vi "main.vi"() -> ()   [LabVIEW 2019]
uses:
  ServerCommands.ctl
  <vilib>/ErrorRing/Error Ring.xnode
panel:
  out "Log":string
  in  "stop":bool
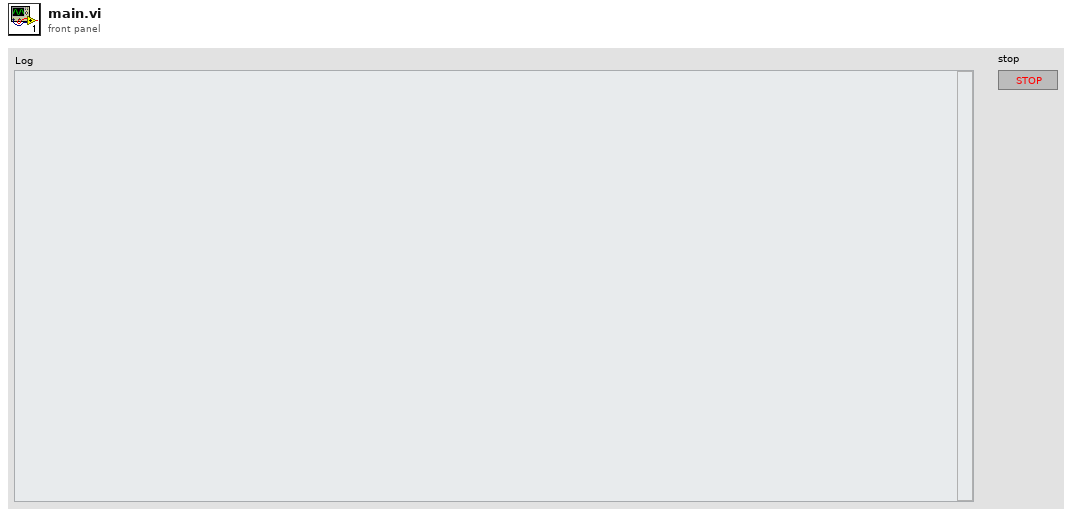
[diagram p1: front panel]
types:
  T1 = typedef "ServerCommands.ctl" = enum16{"Initialize", "Listen", "Run"}
  T2 = enum16{"Standard", "Buffered", "CRLF", "Immediate"}
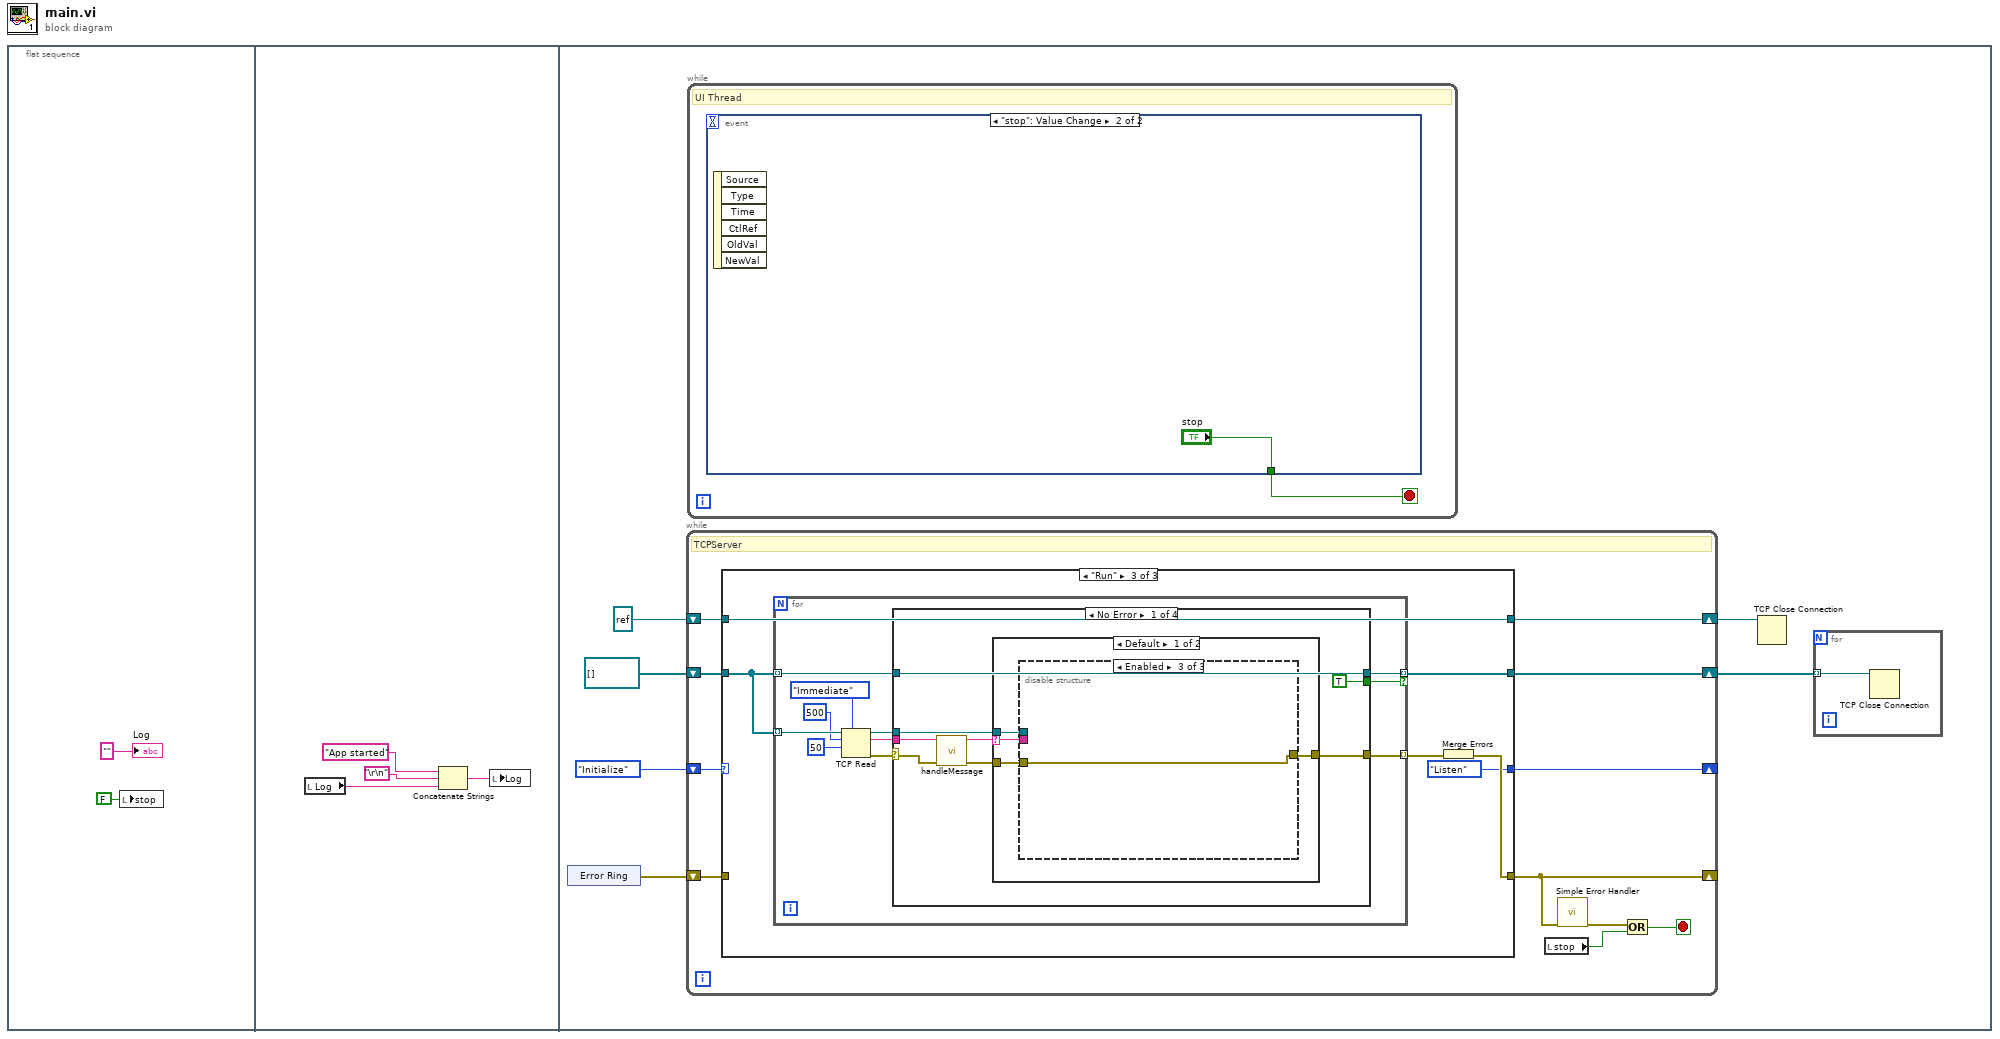
[diagram p0: block diagram]
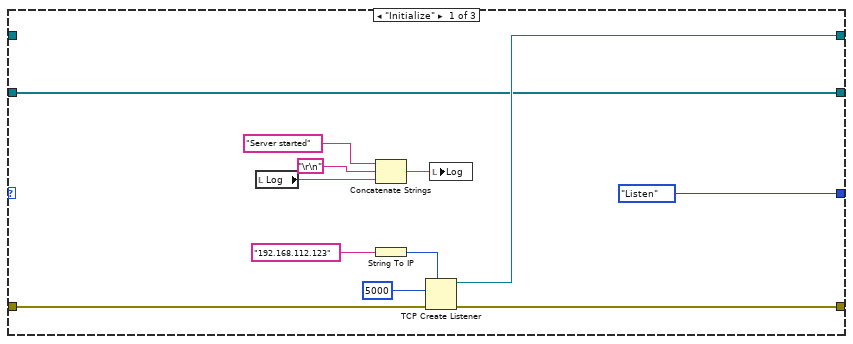
[diagram p2: hidden frame]
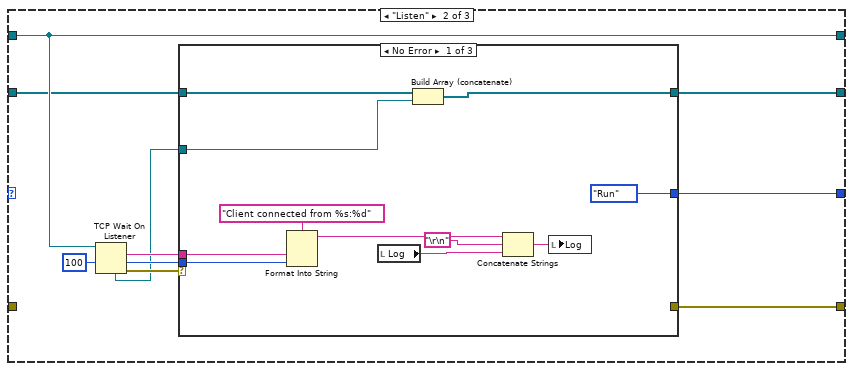
[diagram p3: hidden frame]
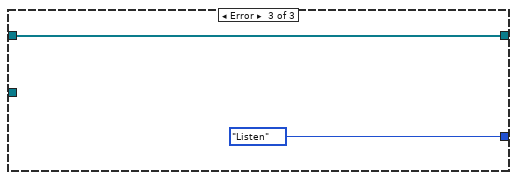
[diagram p5: hidden frame]
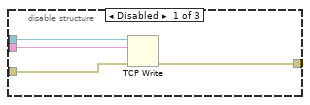
[diagram p6: hidden frame]
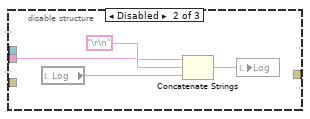
[diagram p7: hidden frame]
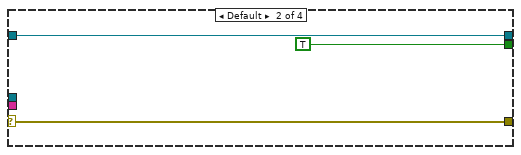
[diagram p9: hidden frame]
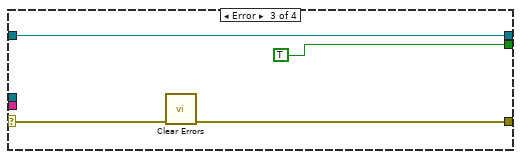
[diagram p10: hidden frame]
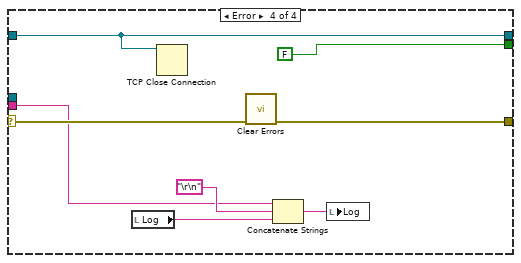
[diagram p11: hidden frame]
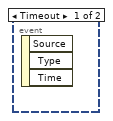
[diagram p12: hidden frame]
diagram:
  n1 = flat-sequence {
    frame #0 {
      n2 = local write "stop"(FALSE ("stop")) -> ()
      "Log" <- ""
    }
    frame #1 {
      n3 = local read "Log"() -> (w6:string)
      n4 = Concatenate Strings("App started" ("string"), "\r\n", w6) -> (w5:string)
      n5 = local write "Log"(w5) -> ()
    }
    frame #2 {
      n6 = xnode "Error Ring"() -> ("error out"=w11:errorcluster)
      n7 = while {
        shift-right: [w20] -> _
        shift-left: w11 -> [w24]
        shift-right: [w22] -> w8
        shift-left: refnum<k5> refnum ("listener ID") -> [w23]
        shift-right: [w21] -> _
        shift-left: ServerCommands."Initialize" ("ServerCommands") -> [w25]
        shift-right: [w15] -> w7
        shift-left: refnum<k5>[] [] -> [w16]
        stop <- w17 stop-if-true
        # "TCPServer"
        n8 = case shown="\"Run\"" w25 {
          tunnel: w24 -> [w33 _ _]
          tunnel: [w34 w43 w67] -> w20
          tunnel: [w32 w47 w68] -> w22
          tunnel: w23 -> [_ w47 w68]
          tunnel: [ServerCommands."Listen" ("ServerCommands") w41 ServerCommands."Listen" ("ServerCommands")] -> w21
          tunnel: w16 -> [w26 w40 w65]
          tunnel: [w26 w39 w64] -> w15
          frame "Initialize" {
            n9 = local read "Log"() -> (w29:string)
            n10 = Concatenate Strings("Server started" ("string"), "\r\n", w29) -> (w27:string)
            n11 = String To IP(1:"192.168.112.123" ("name")) -> (0:w37:u32)
            n12 = TCP Create Listener(7:w37, 8:w33, 10:u16 5000 ("port")) -> (0:w34:errorcluster, 3:w32:refnum<k5>)  [unwired: 2 in, 1 out]
            n13 = local write "Log"(w27) -> ()
          }
          frame "Listen" {
            n14 = TCP Wait On Listener(9:100 ("timeout ms (wait forever: -1)"), 11:w47) -> (0:w46:errorcluster, 1:w44:u16, 2:w45:string, 4:w38:refnum<k5>)  [unwired: 2 in, 1 out]
            n15 = case shown="No Error" w46 {
              selector: w46 -> [_ w60 _]
              tunnel: w38 -> [w49 _ _]
              tunnel: w45 -> [w54 _ _]
              tunnel: w44 -> [w53 _ _]
              tunnel: [_ w60 _] -> w43
              tunnel: [ServerCommands."Run" ("ServerCommands") _ ServerCommands."Listen" ("ServerCommands")] -> w41
              tunnel: w40 -> [w50 w59 w61]
              tunnel: [w48 w59 w61] -> w39
              frame No Error {
                n16 = Format Into String(format string="Client connected from %s:%d", w54, w53) -> (resulting string=w52:string)  [unwired: 2 in, 1 out]
                n17 = local read "Log"() -> (w56:string)
                n18 = Build Array (concatenate)(w50, w49) -> (w48:refnum<k5>[])
                n19 = Concatenate Strings(w52, "\r\n", w56) -> (w57:string)
                n20 = local write "Log"(w57) -> ()
              }
              frame Default {
              }
              frame Error {
              }
            }
          }
          frame "Run" {
            n21 = for {
              tunnel: w65 -> [w79] mode=indexing
              tunnel: [w74] -> w66 mode=indexing
              tunnel: w65 -> [w73] mode=indexing
              tunnel: [w72] -> w64 mode=indexing if=w71
              n22 = TCP Read(connection ID=w79, bytes to read=500, 7:T2."Immediate" ("mode (standard)"), 9:50 ("timeout ms (25000)")) -> (connection ID out=w75:refnum<k5>, data out=w76:string, error out=w77:errorcluster)  [unwired: 1 in]
              n23 = case shown="No Error" w77 {
                selector: w77 -> [w86 w104 w108 w116]
                tunnel: w76 -> [w87 _ _ w109]
                tunnel: w75 -> [w83 _ _ _]
                tunnel: [w82 w104 w107 w115] -> w74
                tunnel: w73 -> [w81 w103 w106 w113]
                tunnel: [w81 w103 w106 w113] -> w72
                tunnel: [TRUE TRUE TRUE FALSE] -> w71
                frame No Error {
                  n24 = call "handleMessage.vi"("error in (no error)"=w86, "InputMessage"=w87) -> ("error out"=w84:errorcluster, "OutputMessage"=w85:string)  [unwired: 8 in]
                  n25 = case shown="Default" w85 {
                    selector: w85 -> [w90 _]
                    tunnel: w84 -> [w89 w101]
                    tunnel: w83 -> [w91 _]
                    tunnel: [w88 w101] -> w82
                    frame Default {
                      n26 = disable-structure shown="Enabled" {
                        disable-tunnel: w91 -> [w95 _ _]
                        disable-tunnel: w90 -> [w94 w96 _]
                        disable-tunnel: w89 -> [w93 _ w100]
                        disable-tunnel: [w92 _ w100] -> w88
                        frame Disabled {
                          n27 = TCP Write(connection ID=w95, data in=w94, error in (no error)=w93) -> (error out=w92:errorcluster)  [unwired: 1 in, 2 out]
                        }
                        frame Disabled {
                          n28 = local read "Log"() -> (w97:string)
                          n29 = Concatenate Strings(w96, "\r\n", w97) -> (w98:string)
                          n30 = local write "Log"(w98) -> ()
                        }
                        frame Enabled {
                        }
                      }
                    }
                    frame "" {
                    }
                  }
                }
                frame Default {
                }
                frame Error {
                  n31 = call <vilib>:"Clear Errors.vi"("error in (no error)"=w108) -> ("error out"=w107:errorcluster)  [unwired: 5 in, 1 out]
                }
                frame Error {
                  n32 = local read "Log"() -> (w111:string)
                  n33 = TCP Close Connection(connection ID=w113) -> ()  [unwired: 2 in, 2 out]
                  n34 = call <vilib>:"Clear Errors.vi"("error in (no error)"=w116) -> ("error out"=w115:errorcluster)  [unwired: 5 in, 1 out]
                  n35 = Concatenate Strings(w109, "\r\n", w111) -> (w112:string)
                  n36 = local write "Log"(w112) -> ()
                }
              }
            }
            n37 = Merge Errors(w66) -> (w67:errorcluster)
          }
        }
        n38 = local read "stop"() -> (w18:bool)
        n39 = call <vilib>:"Simple Error Handler.vi"("error in (no error)"=w20) -> ("error out"=w19:errorcluster)  [unwired: 4 in, 4 out]
        n40 = Or(x=w19, y=w18) -> (x .or. y?=w17:bool)
      }
      n41 = while {
        stop <- w117 stop-if-true
        # "UI Thread"
        n42 = event shown="[1] \"stop\": Value Change" {
          selector: _ -> [_ _]
          dyn-events: _ -> [_ _]
          timeout: _ -> [_ _]
          tunnel: [_ "stop"] -> w117
          event Timeout {
            n43 = event-data() -> ()  [unwired: 1 in, 3 out]
          }
          event "stop": Value Change {
            n44 = event-data() -> ()  [unwired: 1 in, 6 out]
          }
        }
      }
      n45 = TCP Close Connection(connection ID=w8) -> ()  [unwired: 2 in, 2 out]
      n46 = for {
        tunnel: w7 -> [w13] mode=indexing
        n47 = TCP Close Connection(connection ID=w13) -> ()  [unwired: 2 in, 2 out]
      }
    }
  }
